vi "from string array.vi"(8 "error in (no error)":errorcluster, 9 "String Array":string[][](array[string]), 10 "version":string, 11 "module configuration in":refnum<class "Scan Engine configuration.lvclass">) -> (0 "error out":errorcluster, 3 "module configuration out":refnum<class "Scan Engine configuration.lvclass">)   [LabVIEW 2015, in "Scan Engine configuration.lvclass"]
uses:
  Scan Engine configuration.lvclass
  Line.ctl
  <vilib>/NI/Tag Bus Module Framework/channel/TBM channel.lvclass
  permissions.ctl
  <vilib>/NI/Tag Bus/tag/Data Type.ctl
  Scan Engine configuration.lvclass/Scan Engine configuration.ctl
  Write Lines.vi
  Get Line Name.vi
  Find Duplicate.vi
  <vilib>/Utility/error.llb/Error Cluster From Error Code.vi
  <vilib>/NI/Tag Bus/tag/tag descriptor.lvclass
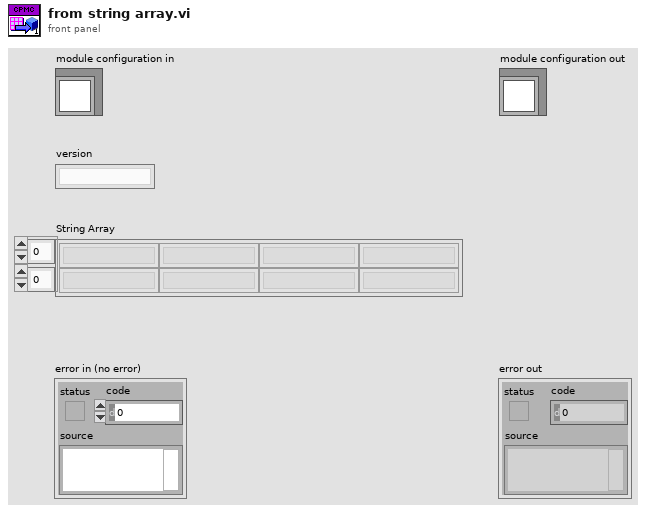
[diagram p1: front panel]
types:
  T1 = typedef "tag bus.lvlib/tag descriptor.lvclass/Data Type.ctl" = enum16{"Double", "Single", "I64", "I32", "I16", "I8", "U64", "U32", "U16", "U8", "Boolean", "String", "Array of Double", "Array of Single", "Array of I64", "Array of I32", "Array of I16", "Array of I8", "Array of U64", "Array of U32", "Array of U16", "Array of U8", "Array of Boolean", "Array of String"}
  T2 = typedef "Scan Engine configuration.lvclass/permissions.ctl" = enum32{"Read from HW", "Write to HW"}
  T3 = typedef "Scan Engine configuration.lvclass/Line.ctl" = cluster{"channel":refnum<class "TBM channel.lvclass">, "Tag":string}
  T4 = typedef "TBM channel.lvclass/channel classification.ctl" = enum16{"input data", "output data", "processing parameter", "processing result"}
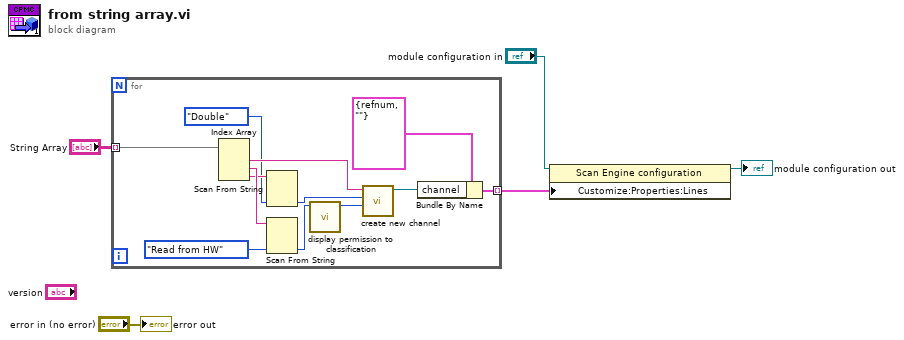
[diagram p0: block diagram]
diagram:
  n1 = for {
    tunnel: [w16] -> w2 mode=indexing
    tunnel: "String Array" -> [w15] mode=indexing
    n2 = Index Array(array=w15) -> (element #1=w13:string, element #2=w12:string, element #3=w11:string)  [unwired: 3 in]
    n3 = Scan From String(input string=w11, default 1=Data_Type."Double" ("data type")) -> (output 1=w6:T1)  [unwired: 3 in, 3 out]
    n4 = Scan From String(input string=w12, default 1=permissions."Read from HW" ("display permissions")) -> (output 1=w9:T2)  [unwired: 3 in, 3 out]
    n5 = call "display permission to classification.vi"("display permissions"=w9) -> ("channel classification"=w8:T4)  [unwired: 10 in]
    n6 = call <vilib>:"create new channel.vi"("channel classification"=w8, "data type"=w6, "channel name"=w13) -> ("channel"=w14:refnum<class "TBM channel.lvclass">)  [unwired: 8 in]
    n7 = Bundle By Name(cluster=T3 {"channel"=refnum, "Tag"=""} ("Line"), "channel"=w14) -> (w16:T3)
  }
  n8 = property class="Scan Engine configuration"(reference="module configuration in", "Customize:Properties:Lines"=w2) -> (reference out=→"module configuration out":refnum<class "Scan Engine configuration.lvclass">)  [unwired: 1 in, 1 out]
  "error out" <- "error in (no error)"
